vi "Test.vi"() -> ()   [LabVIEW 2019]
panel:
  out "data out 2":string
  out "data out":string
  in  "Beam":bool
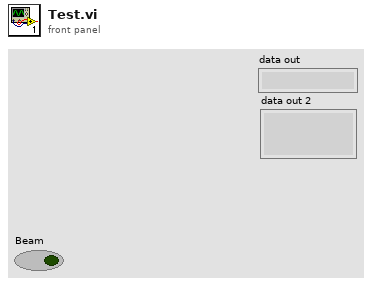
[diagram p1: front panel]
types:
  T1 = enum16{"Standard", "Buffered", "CRLF", "Immediate"}
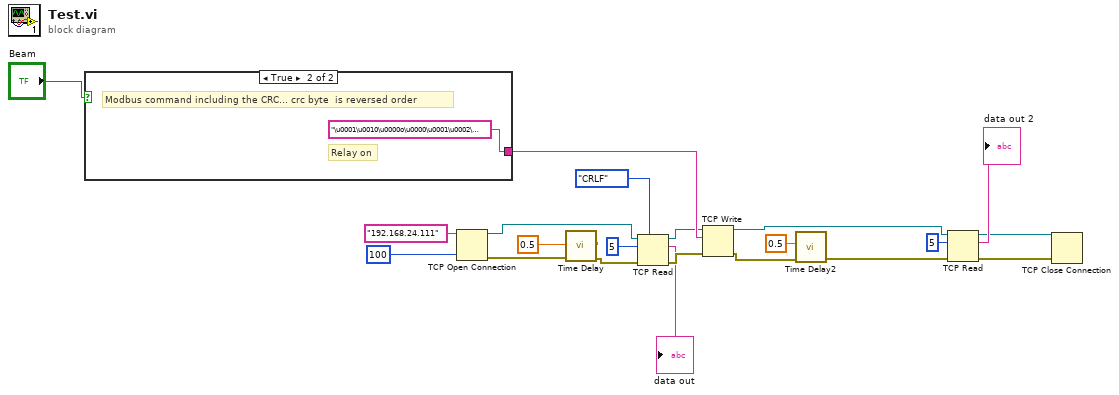
[diagram p0: block diagram]
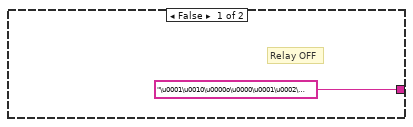
[diagram p2: hidden frame]
diagram:
  n1 = case shown="True" "Beam" {
    tunnel: ["\u0001\u0010\u0000o\u0000\u0001\u0002\u0000\u0000¯\u000f" ("write buffer") "\u0001\u0010\u0000o\u0000\u0001\u0002\u0000\u0001nÏ" ("write buffer")] -> w19
    frame False {
      # "Relay OFF"
    }
    frame True {
      # "Modbus command including the CRC... crc byte  is reversed order"
      # "Relay on"
    }
  }
  n2 = TCP Open Connection(address="192.168.24.111", remote port or service name=u16 100) -> (connection ID=w10:refnum<k5>, error out=w21:errorcluster)  [unwired: 3 in]
  n3 = call "Time Delay"("error in (no error)"=w21, "Delay Time (s)"=0.5) -> ("error out"=w13:errorcluster)  [unwired: 9 in]
  n4 = TCP Read(connection ID=w10, bytes to read=5, error in (no error)=w13, 7:T1."CRLF" ("mode (standard)")) -> (connection ID out=w11:refnum<k5>, data out=→"data out":string, error out=w12:errorcluster)  [unwired: 1 in]
  n5 = TCP Write(connection ID=w11, data in=w19, error in (no error)=w12) -> (connection ID out=w4:refnum<k5>, error out=w18:errorcluster)  [unwired: 1 in, 1 out]
  n6 = call "Time Delay2"("error in (no error)"=w18, "Delay Time (s)"=0.5) -> ("error out"=w6:errorcluster)  [unwired: 9 in]
  n7 = TCP Read(connection ID=w4, bytes to read=5, error in (no error)=w6) -> (connection ID out=w1:refnum<k5>, data out=→"data out 2":string, error out=w5:errorcluster)  [unwired: 2 in]
  n8 = TCP Close Connection(connection ID=w1, error in (no error)=w5) -> ()  [unwired: 1 in, 2 out]
